vi "Load State Data.vi"(8 "error in (no error)":errorcluster, 11 "Calendar in":refnum<class "Calendar.lvclass">) -> (0 "error out":errorcluster, 3 "Calendar out":refnum<class "Calendar.lvclass">)   [LabVIEW 2020, in "Calendar.lvclass"]
doc: "The <b>Load State Data VI</b> is a dynamic dispatch VI that must be overwritten in every QControl Class that uses the State Data. If used it must <b>Call Parent Method</b>. This recursively loads the Data Value Reference to the data space for the QControl Class up the inheritance hierarchy that uses the Data Value Reference.\n<b> </b> <b> </b>\n©2016 Q Software Innovations, LLC (QSI)\nwritten by Quentin Alldredge\nproduced in LabVIEW 2015\n\nsupport@qsoftwareinnovations.com\nwww.qsoftwareinnovations.com\n\nAll rights reserved.\n\nRedistribution and use in source and binary forms, with or without modification, are permitted provided that the following conditions are met:\n\n * Redistributions of source code must retain the above copyright notice, this list of conditions and the following disclaimer.\n * Redistributions in binary form must reproduce the above copyright notice, this list of conditions and the following disclaimer in the documentation and/or other materials provided with the distribution.\n * Neither the name of Q Software Innovations, LLC. nor the names of its contributors may be used to endorse or promote products derived from this software without specific prior written permission.\n\nTHIS SOFTWARE IS PROVIDED BY THE COPYRIGHT HOLDERS AND CONTRIBUTORS \"AS IS\" AND ANY EXPRESS OR IMPLIED WARRANTIES, INCLUDING, BUT NOT LIMITED TO, THE IMPLIED WARRANTIES OF MERCHANTABILITY AND FITNESS FOR A PARTICULAR PURPOSE ARE DISCLAIMED. IN NO EVENT SHALL THE COPYRIGHT OWNER OR CONTRIBUTORS BE LIABLE FOR ANY DIRECT, INDIRECT, INCIDENTAL, SPECIAL, EXEMPLARY, OR CONSEQUENTIAL DAMAGES (INCLUDING, BUT NOT LIMITED TO, PROCUREMENT OF SUBSTITUTE GOODS OR SERVICES; LOSS OF USE, DATA, OR PROFITS; OR BUSINESS INTERRUPTION) HOWEVER CAUSED AND ON ANY THEORY OF LIABILITY, WHETHER IN CONTRACT, STRICT LIABILITY, OR TORT (INCLUDING NEGLIGENCE OR OTHERWISE) ARISING IN ANY WAY OUT OF THE USE OF THIS SOFTWARE, EVEN IF ADVISED OF THE POSSIBILITY OF SUCH DAMAGE."
uses:
  Calendar.lvclass
  State Data.ctl
  DaysOfWeek.ctl
  Calendar.lvclass/Calendar.ctl
  <vilib>/QSI/QControls/QControl Classes/Cluster/Cluster.lvclass
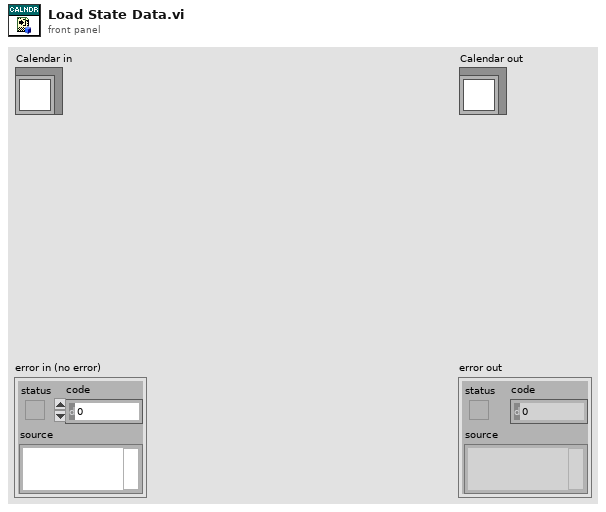
[diagram p1: front panel]
types:
  T1 = typedef "Calendar.lvclass/DaysOfWeek.ctl" = enum16{"Sunday", "Monday", "Tuesday", "Wednesday", "Thursday", "Friday", "Saturday"}
  T2 = typedef "Calendar.lvclass/State Data.ctl" = cluster{"Current Date":timestamp, "First Day of Week":T1, "Color":cluster{"Selector Background":u32, "Selector Text":u32, "Days of Week Background":u32, "Days of Week Text":u32, "Calendar Background":u32, "Calendar Text":u32, "Calendar Selection Background":u32, "Calendar Selection Text":u32}, "Visible":cluster{"Today Selector Visible":bool, "Month-Year Selector Visible":bool}}
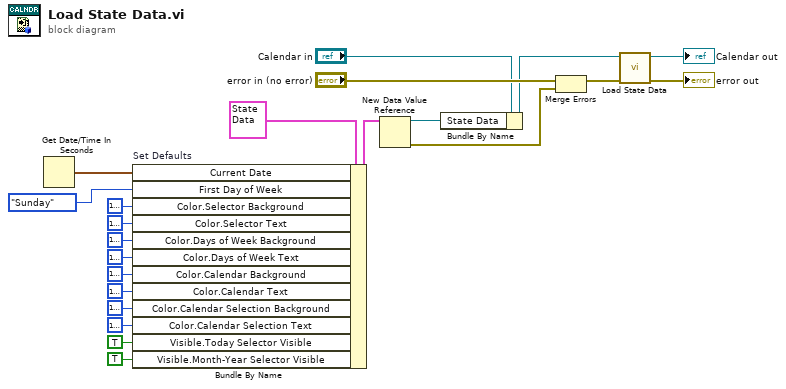
[diagram p0: block diagram]
diagram:
  n1 = Get Date/Time In Seconds() -> (seconds since 1Jan1904=w12:timestamp)
  n2 = Bundle By Name "Set Defaults"(cluster=T2 {"Current Date"=timestamp(0 s since 1904-01-01), "First Day of Week"=enum."Sunday", "Color"={"Selector Background"=0, "Selector Text"=0, "Days of Week Background"=0, "Days of Week Text"=0, "Calendar Background"=0, "Calendar Text"=0, "Calendar Selection Background"=0, "Calendar Selection Text"=0}, "Visible"={"Today Selector Visible"=FALSE, "Month-Year Selector Visible"=FALSE}} ("State Data"), "Current Date"=w12, "First Day of Week"=DaysOfWeek."Sunday", "Color.Selector Background"=u32 16777238, "Color.Selector Text"=u32 16777222, "Color.Days of Week Background"=u32 16777238, "Color.Days of Week Text"=u32 16777222, "Color.Calendar Background"=u32 16777226, "Color.Calendar Text"=u32 16777222, "Color.Calendar Selection Background"=u32 16777224, "Color.Calendar Selection Text"=u32 16777225, "Visible.Today Selector Visible"=TRUE, "Visible.Month-Year Selector Visible"=TRUE) -> (w13:T2)
  n3 = New Data Value Reference(data value=w13) -> (data value reference=w17:refnum<data-value>, error out=w15:errorcluster)  [unwired: 1 in]
  n4 = Bundle By Name(cluster="Calendar in", "State Data"=w17) -> (w18:refnum<class "Calendar.lvclass">)
  n5 = Merge Errors("error in (no error)", w15) -> (w16:errorcluster)
  n6 = call-parent "Load State Data.vi"("error in (no error)"=w16, "Control in"=w18) -> ("error out"=→"error out":errorcluster, "Control out"=→"Calendar out":refnum<class "Calendar.lvclass">)  [unwired: 8 in]
